vi "Double2WaveWithFlag2 Signals.vi"(1 "Input 2":dbl[](array[numeric]), 2 "Input 1":dbl[](array[numeric]), 3 "Index Flag":bool[](array[boolean]) caption="Flag") -> (0 "Waveform Chart":waveform(dbl)[](graph))   [LabVIEW 2009]
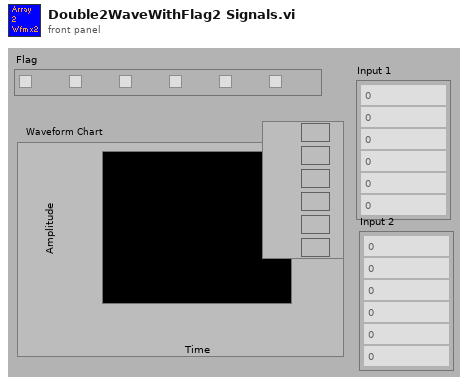
[diagram p1: front panel]
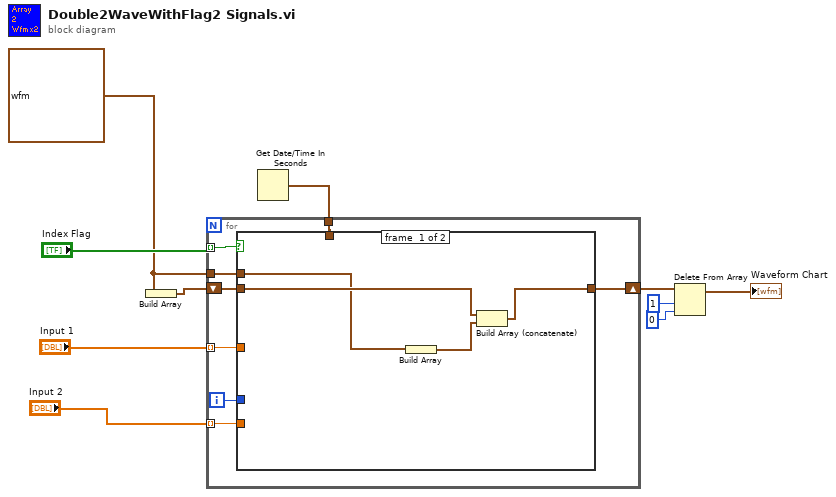
[diagram p0: block diagram]
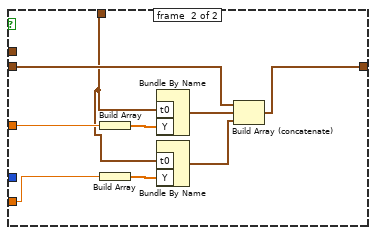
[diagram p2: hidden frame]
diagram:
  w2 = waveform(dbl) {"t0"=timestamp(0 s since 1904-01-01), "dt"=1.0, "Y"=[]} ("waveform A 2")
  n1 = Build Array(w2) -> (w7:waveform(dbl)[])
  n2 = Get Date/Time In Seconds() -> (seconds since 1Jan1904=w10:timestamp)
  n3 = for {
    tunnel: "Index Flag" -> [w18] mode=indexing
    shift-right: [w15] -> w6
    shift-left: w7 -> [w16]
    tunnel: w10 -> [w14]
    tunnel: "Input 1" -> [w13] mode=indexing
    tunnel: w2 -> [w12]
    tunnel: "Input 2" -> [w11] mode=indexing
    i -> [w17]
    n4 = case shown="True" w18 {
      tunnel: w17 -> [_ _]
      tunnel: w16 -> [w21 w27]
      tunnel: [w20 w28] -> w15
      tunnel: w14 -> [_ w24]
      tunnel: w13 -> [_ w29]
      tunnel: w12 -> [w19 _]
      tunnel: w11 -> [_ w25]
      frame #0 {
        n5 = Build Array(w19) -> (w22:waveform(dbl)[])
        n6 = Build Array (concatenate)(w21, w22) -> (w20:waveform(dbl)[])
      }
      frame #1 {
        n7 = Build Array(w29) -> (w30:dbl[])
        n8 = Build Array(w25) -> (w26:dbl[])
        n9 = Bundle By Name("t0"=w24, "Y"=w30) -> (w31:waveform(dbl))  [unwired: 1 out]
        n10 = Bundle By Name("t0"=w24, "Y"=w26) -> (w23:waveform(dbl))  [unwired: 1 out]
        n11 = Build Array (concatenate)(w27, w31, w23) -> (w28:waveform(dbl)[])
      }
    }
  }
  n12 = Delete From Array(array=w6, length=1, index=0) -> (array with subset deleted=→"Waveform Chart":waveform(dbl)[])  [unwired: 1 out]
